vi "1D DBL To Config String.vi"(5 "Digit":u32=6, 7 "Interval":string=",", 10 "Array In":dbl[](array[numeric]) format="%#_f") -> (2 "String Out":string)   [LabVIEW 2024]
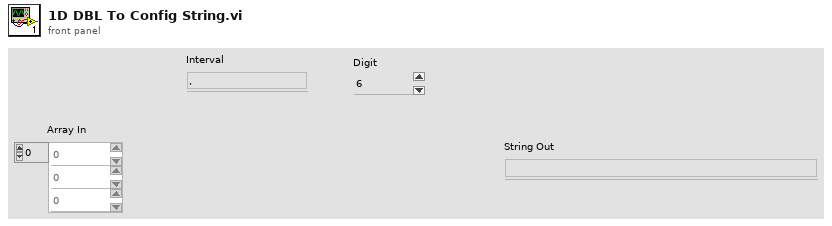
[diagram p1: front panel]
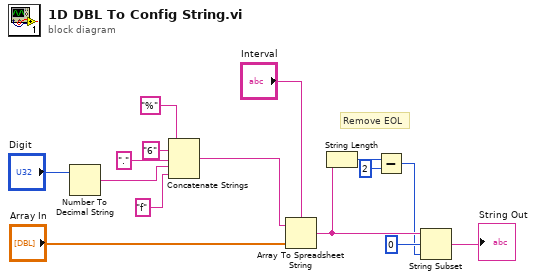
[diagram p0: block diagram]
diagram:
  # "Remove EOL"
  n1 = Number To Decimal String(number="Digit") -> (decimal integer string=w2:string)  [unwired: 1 in]
  n2 = Concatenate Strings("%" ("string"), "6" ("string"), "." ("string"), w2, "f" ("string")) -> (w5:string)
  n3 = Array To Spreadsheet String(delimiter (Tab)="Interval", array="Array In", 3:w5) -> (spreadsheet string=w14:string)
  n4 = String Length(string=w14) -> (length=w13:i32)
  n5 = Subtract(x=w13, y=2) -> (x-y=w10:i32)
  n6 = String Subset(string=w14, offset (0)=0, length (rest)=w10) -> (substring=→"String Out":string)
